vi "Configure Measurement (Adjacent Channel Power Ratio).vi"(0 "VISA resource name":refnum<visa-resource-name>, 5 "Integration Range (1E+6 Hz)":i32=1000000, 9 "Center Frequency (3.5E+9 Hz)":dbl=3500000000.0, 11 "error in (no error)":errorcluster) -> (4 "VISA resource name out":refnum<visa-resource-name>, 15 "error out":errorcluster)   [LabVIEW 2022 SP3, in "Agilent N934X Series.lvlib"]
doc: "Sets the Adjacent Channel Power Ratio measurement parameters."
uses:
  <instrlib>/Agilent N934X Series/Agilent N934X Series.lvlib
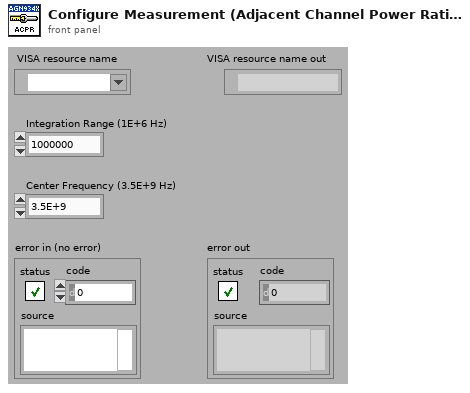
[diagram p1: front panel]
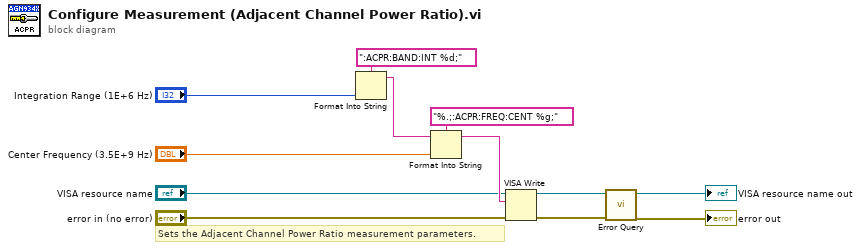
[diagram p0: block diagram]
diagram:
  # "Sets the Adjacent Channel Power Ratio measurement parameters."
  n1 = Format Into String(format string=":ACPR:BAND:INT %d;", "Integration Range (1E+6 Hz)") -> (resulting string=w10:string)  [unwired: 2 in, 1 out]
  n2 = Format Into String(format string="%.;:ACPR:FREQ:CENT %g;", initial string=w10, "Center Frequency (3.5E+9 Hz)") -> (resulting string=w7:string)  [unwired: 1 in, 1 out]
  n3 = VISA Write(VISA resource name="VISA resource name", write buffer=w7, error in (no error)="error in (no error)") -> (VISA resource name out=w4:refnum<visa-resource-name>, error out=w3:errorcluster)  [unwired: 1 out]
  n4 = call <instrlib>:"Error Query.vi"("error in (no error)"=w3, "VISA resource name"=w4) -> ("error out"=→"error out":errorcluster, "VISA resource name out"=→"VISA resource name out":refnum<visa-resource-name>)  [unwired: 6 in, 2 out]
